vi "Event-眼球轉動.vi"() -> ()   [LabVIEW 2019]
uses:
  Eye.ctl
panel:
  in  "stop":bool
  out "Eye":T1 scale=0.0..10.0
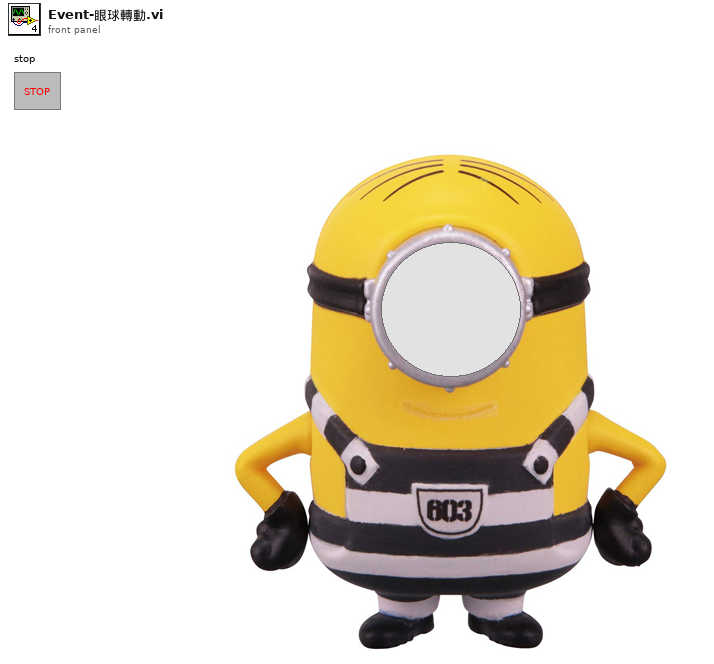
[diagram p1: front panel]
types:
  T1 = typedef "Eye.ctl" = dbl
  T2 = typedef "LVBoundsTypeDef.ctl" = cluster{"Width":u32, "Height":u32}
  T3 = typedef "LVPositionTypeDef.ctl" = cluster{"Left":i32, "Top":i32}
  T4 = typedef "LVPoint32TypeDef.ctl" = cluster{"Horizontal":i32, "Vertical":i32}
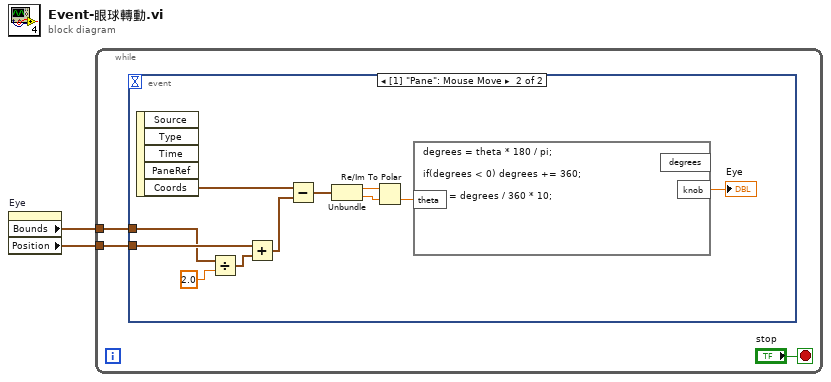
[diagram p0: block diagram]
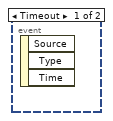
[diagram p2: hidden frame]
diagram:
  n1 = property on="Eye" class="Knob (strict)"() -> ("Bounds"=w2:T2, "Position"=w1:T3)  [unwired: 2 in, 2 out]
  n2 = while {
    tunnel: w2 -> [w4]
    tunnel: w1 -> [w3]
    stop <- "stop" stop-if-true
    n3 = event shown="[1] \"Pane\": Mouse Move" {
      selector: _ -> [_ _]
      dyn-events: _ -> [_ _]
      timeout: _ -> [_ _]
      tunnel: w4 -> [_ w15]
      tunnel: w3 -> [_ w16]
      event Timeout {
        n4 = event-data() -> ()  [unwired: 1 in, 3 out]
      }
      event Mouse Move {
        n5 = event-data() -> ("Coords"=w12:T4)  [unwired: 1 in, 4 out]
        n6 = Divide(x=w15, y=2.0) -> (x/y=w13:cluster{"Width":dbl, "Height":dbl})
        n7 = Add(x=w16, y=w13) -> (x+y=w11:cluster{dbl, dbl})
        n8 = Subtract(x=w12, y=w11) -> (x-y=w10:cluster{dbl, dbl})
        n9 = Unbundle(w10) -> (w9:dbl, w8:dbl)
        n10 = Re/Im To Polar(2:w8, 3:w9) -> (0:w7:dbl)  [unwired: 1 out]
        n11 = formula code="degrees = theta * 180 / pi;\n\nif(degrees < 0) degrees += 360;\n\nknob = degrees / 360 * 10;"("theta"=w7) -> ("knob"=→"Eye":dbl)  [unwired: 1 out]
      }
    }
  }
